vi "need for local2.vi"() -> ()   [LabVIEW 2013]
panel:
  in  "stop":bool
  out "Loop 2 executed":bool
  in  "ON/OFF":bool
  out "Loop 1 executed":bool
  in  "ON/OFF":bool
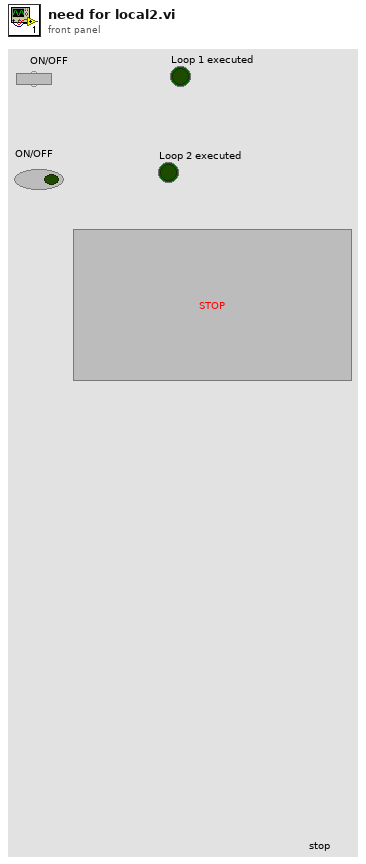
[diagram p1: front panel]
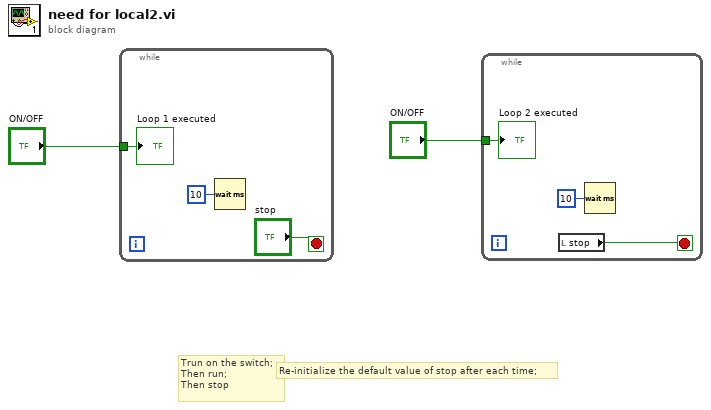
[diagram p0: block diagram]
diagram:
  # "Re-initialize the default value of stop after each time;"
  # "Trun on the switch;\nThen run;\nThen stop"
  n1 = while {
    tunnel: "ON/OFF" -> [w5]
    stop <- "stop" stop-if-true
    n2 = Wait (ms)(milliseconds to wait=u32 10) -> ()  [unwired: 1 out]
    "Loop 1 executed" <- w5
  }
  n3 = while {
    tunnel: "ON/OFF" -> [w8]
    stop <- w6 stop-if-true
    n4 = local read "stop"() -> (w6:bool)
    n5 = Wait (ms)(milliseconds to wait=u32 10) -> ()  [unwired: 1 out]
    "Loop 2 executed" <- w8
  }
